vi "Rectangle Apply Inkscape Ratio.vi"(1 "rects in":T2(array[cluster])) -> (0 "rects out":T2(array[cluster]))   [LabVIEW 2019]
uses:
  <vilib>/Analysis/Matrix/Datatypes/RealMatrix.ctl
  Global Variables.vi
  <vilib>/Analysis/Matrix/NI_Matrix.lvlib
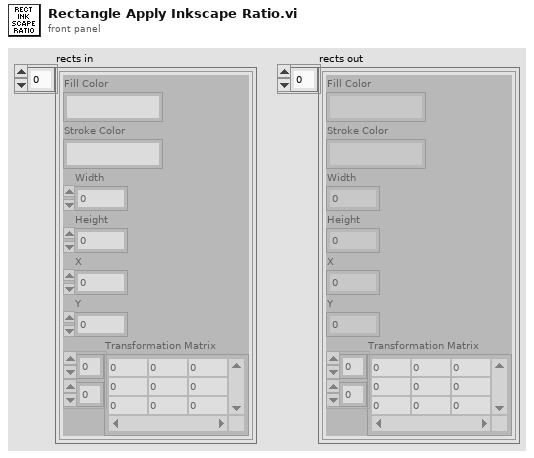
[diagram p1: front panel]
types:
  T1 = typedef "NI_Matrix.lvlib/RealMatrix.ctl" = dbl[][]
  T2 = cluster{"Fill Color":string, "Stroke Color":string, "Width":dbl, "Height":dbl, "X":dbl, "Y":dbl, "Transformation Matrix":T1}[]
  T3 = cluster{"Fill Color":string, "Stroke Color":string, "Width":dbl, "Height":dbl, "X":dbl, "Y":dbl, "Transformation Matrix":T1}
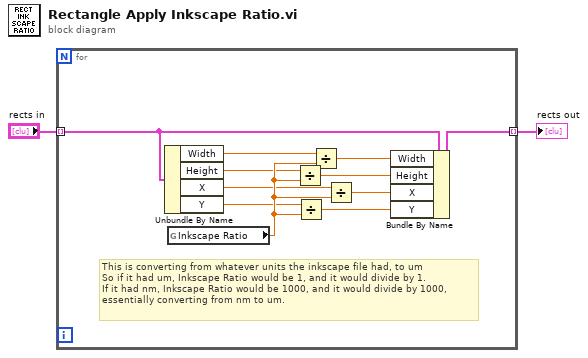
[diagram p0: block diagram]
diagram:
  n1 = for {
    tunnel: "rects in" -> [w7] mode=indexing
    tunnel: [w6] -> w2 mode=indexing
    # "This is converting from whatever units the inkscape file had, to um\nSo if it had um, Inkscape Ratio would be 1, and it would divide by 1.\nIf it had nm, Inkscape Ratio would be 1000, and it would divide by 1000,\nessentially converting from nm to um."
    n2 = Unbundle By Name(w7) -> ("Width"=w12:dbl, "Height"=w11:dbl, "X"=w4:dbl, "Y"=w10:dbl)
    n3 = global read "Global Variables.vi" "Inkscape Ratio"() -> (w13:dbl)
    n4 = Divide(x=w11, y=w13) -> (x/y=w9:dbl)
    n5 = Divide(x=w10, y=w13) -> (x/y=w3:dbl)
    n6 = Divide(x=w12, y=w13) -> (x/y=w5:dbl)
    n7 = Divide(x=w4, y=w13) -> (x/y=w8:dbl)
    n8 = Bundle By Name(cluster=w7, "Width"=w5, "Height"=w9, "X"=w8, "Y"=w3) -> (w6:T3)
  }
  "rects out" <- w2
